vi "Read System Status Ref.vi"(8 "error in (no error)":errorcluster, 11 "System Actor in":refnum<class "System Actor.lvclass">) -> (0 "error out":errorcluster, 2 "System Status Ref":refnum<vi>, 3 "System Actor out":refnum<class "System Actor.lvclass">)   [LabVIEW 2014, in "Robot Actors.lvlib" / "System Actor.lvlib" / "System Actor.lvclass"]
uses:
  System Actor.lvclass
  System Status.ctl
  Command/Command Class/Command Status.ctl
  Command/Command Class/Command States.ctl
  Command Processor/Command Processor Class/Command Processor Status.ctl
  Command Processor/Command Processor Class/Command Processor States.ctl
  System Actor.lvclass/System Actor.ctl
  Command/Command Class/Command.lvclass
  Command Processor/Command Processor Class/Command Processor.lvclass
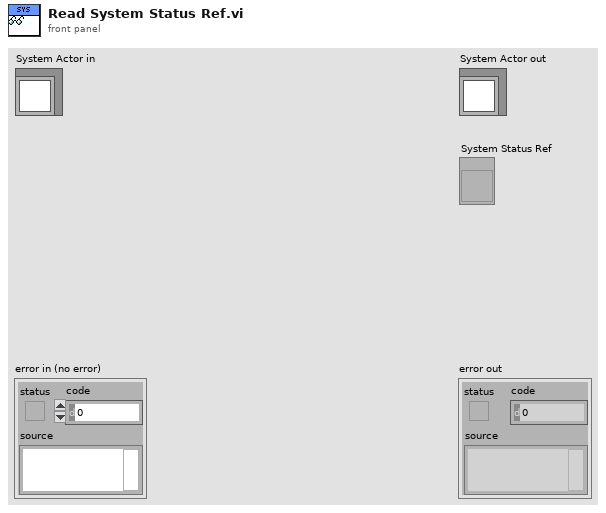
[diagram p1: front panel]
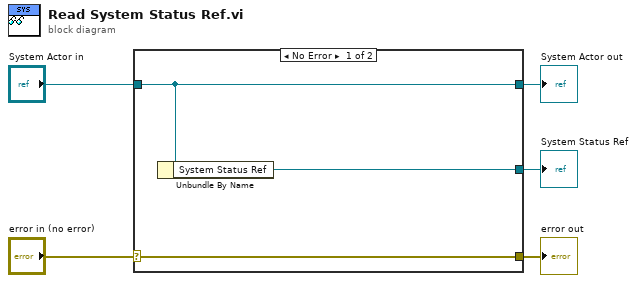
[diagram p0: block diagram]
diagram:
  n1 = case shown="No Error" "error in (no error)" {
    selector: "error in (no error)" -> [w8 w9]
    tunnel: [w8 w9] -> w4
    tunnel: [w7 w10] -> w2
    tunnel: "System Actor in" -> [w7 w10]
    tunnel: [w6 _] -> w1
    frame No Error {
      n2 = Unbundle By Name(w7) -> ("System Status Ref"=w6:refnum<vi>)
    }
    frame Error {
    }
  }
  "error out" <- w4
  "System Actor out" <- w2
  "System Status Ref" <- w1
